vi "Stop Continuous Acquisition.vi"(8 "error in (no error)":errorcluster, 11 "nSensorIP":u32) -> (0 "error out":errorcluster, 3 "function return":i32)   [LabVIEW 2021, in "BonTechDetector.lvlib"]
doc: "extern \"C\" BONTECHLIBRARY_API int __stdcall StopContinuousAcquisition(unsigned int nSensorIP);"
uses:
  BonTechDetector.lvlib
  BonTechWrapperLibrary.dll
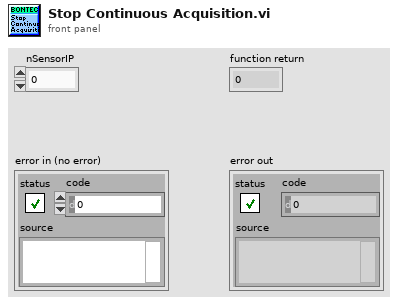
[diagram p1: front panel]
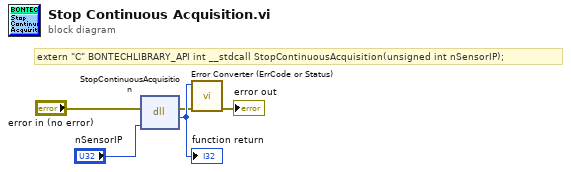
[diagram p0: block diagram]
diagram:
  # "extern \"C\" BONTECHLIBRARY_API int __stdcall StopContinuousAcquisition(unsigned int nSensorIP);"
  n1 = dll-call lib="F:/SourceCodes/ImageHarvest 2021/ImageHandler/BonTechDetector/BonTechWrapperLibrary.dll" fn="StopContinuousAcquisition"(error in="error in (no error)", "nSensorIP"="nSensorIP") -> (error out=w2:errorcluster, "return type"=w5:i32)  [unwired: 3 in, 1 out]
  "function return" <- w5
  n2 = call "Error Converter (ErrCode or Status).vi"("error in (no error)"=w2, "error code"=w5) -> ("error out"=→"error out":errorcluster)  [unwired: 9 in]
